vi "GetAccumulationBlockInfo.vi"(9 "block":T4, 10 "start index":i32, 11 "accumulation settings":T1) -> (1 "condition met":bool, 2 "stop index (include)":i32, 3 "updated accumulation settings":T1, 5 "acquired (pulses)":i32, 7 "acquired (sec)":dbl)   [LabVIEW 2017, in "DataAccumulator.lvlib"]
uses:
  <vilib>/addons/InsightCM/Devices/Shared/Common/DataAccumulator/DataAccumulator.lvlib
  <vilib>/addons/InsightCM/Devices/Shared/Common/DataAccumulator/controls/AccumulationSettings.ctl
  <vilib>/addons/InsightCM/Devices/Shared/Common/DataAccumulator/controls/accumulationType.ctl
  <vilib>/addons/InsightCM/Devices/Shared/Common/DVRBuffer/controls/BufferLocation.ctl
  <vilib>/addons/InsightCM/Devices/Shared/Common/DVRBuffer/controls/DVRElement.ctl
  <vilib>/addons/InsightCM/Devices/Shared/Common/DVRBuffer/DVRBuffer.lvlib
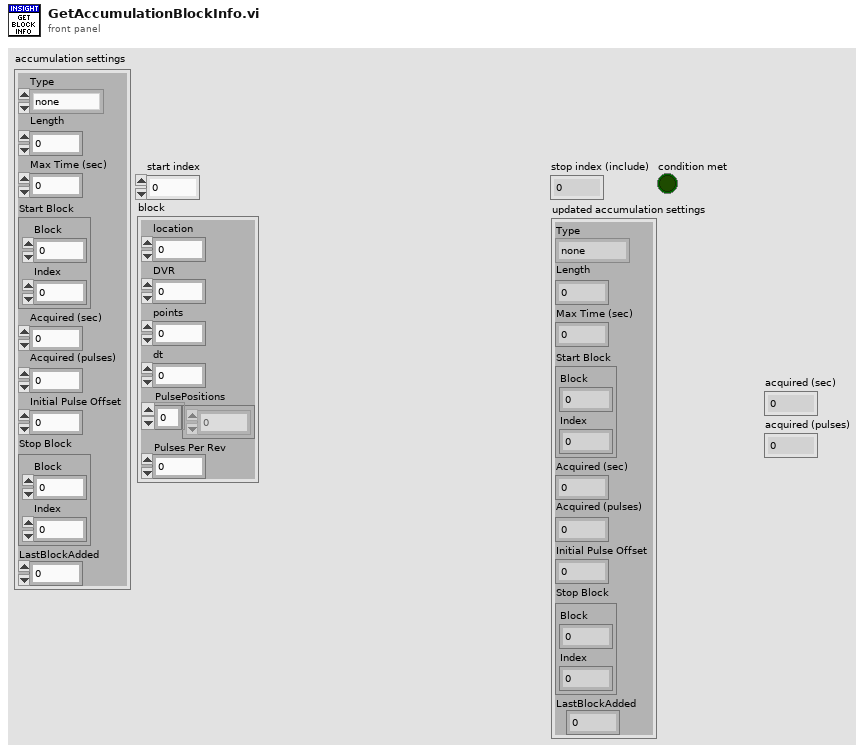
[diagram p1: front panel]
types:
  T1 = typedef "DataAccumulator.lvlib/AccumulationSettings.ctl" = cluster{"Type":T2, "Length":dbl, "Max Time (sec)":dbl, "Start Block":T3, "Acquired (sec)":dbl, "Acquired (pulses)":i32, "Initial Pulse Offset":dbl, "Stop Block":T3, "LastBlockAdded":u32}
  T2 = typedef "DataAccumulator.lvlib/accumulationType.ctl" = enum16{"none", "seconds", "revolutions"}
  T3 = typedef "DVRBuffer.lvlib/BufferLocation.ctl" = cluster{"Block":u32, "Index":i32}
  T4 = typedef "DVRBuffer.lvlib/DVRElement.ctl" = cluster{"location":u32, "DVR":u32, "points":i32, "dt":dbl, "PulsePositions":dbl[], "Pulses Per Rev":dbl}
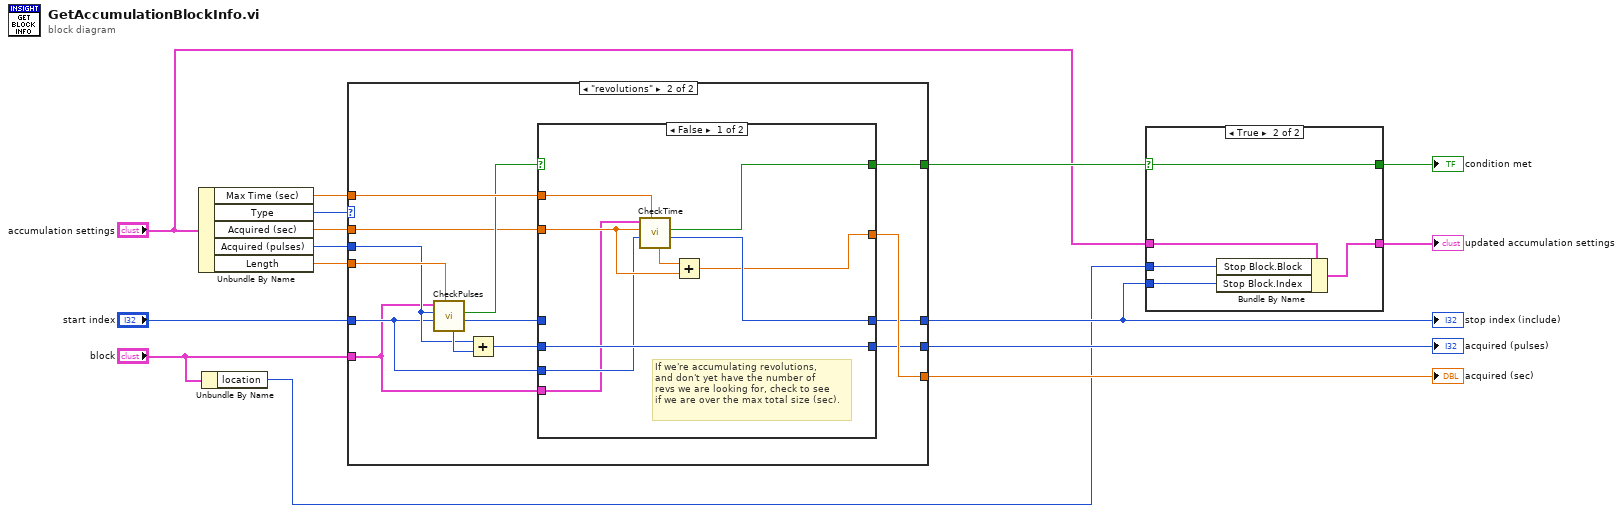
[diagram p0: block diagram]
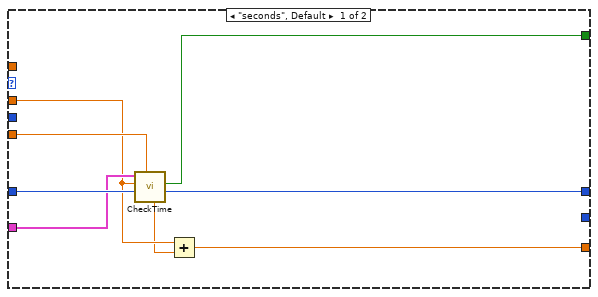
[diagram p3: hidden frame]
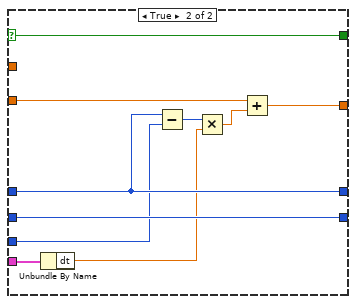
[diagram p4: hidden frame]
diagram:
  n1 = Unbundle By Name("accumulation settings") -> ("Max Time (sec)"=w10:dbl, "Type"=w15:T2, "Acquired (sec)"=w14:dbl, "Acquired (pulses)"=w12:i32, "Length"=w13:dbl)
  n2 = Unbundle By Name("block") -> ("location"=w2:u32)
  n3 = case shown="\"revolutions\"" w15 {
    tunnel: "block" -> [w21 w24]
    tunnel: "start index" -> [w22 w26]
    tunnel: w14 -> [w19 w25]
    tunnel: w13 -> [w20 w37]
    tunnel: [w16 w31] -> w4
    tunnel: [w17 w33] -> w7
    tunnel: [w23 w32] -> w9
    tunnel: w12 -> [_ w35]
    tunnel: w10 -> [_ w34]
    tunnel: [_ w30] -> w8
    frame "seconds", Default {
      n4 = call <vilib>:"CheckTime.vi"("target time"=w20, "start index"=w22, "acquiredSeconds"=w19, "DVR element in"=w21) -> ("stop index (include)"=w16:i32, "time met"=w17:bool, "seconds of data"=w18:dbl)  [unwired: 5 in]
      n5 = Add(x=w19, y=w18) -> (x+y=w23:dbl)
    }
    frame "revolutions" {
      n6 = call <vilib>:"CheckPulses.vi"("target pulses"=w37, "start index"=w26, "acquired pulses in"=w35, "DVR element in"=w24) -> ("stop index (include)"=w27:i32, "pulses met"=w28:bool, "pulses"=w36:i32)  [unwired: 5 in]
      n7 = Add(x=w35, y=w36) -> (x+y=w29:i32)
      n8 = case shown="False" w28 {
        selector: w28 -> [_ w56]
        tunnel: w34 -> [w46 _]
        tunnel: [w45 w56] -> w33
        tunnel: [w41 w52] -> w32
        tunnel: [w44 w51] -> w31
        tunnel: w27 -> [_ w51]
        tunnel: [w43 w55] -> w30
        tunnel: w29 -> [w43 w55]
        tunnel: w26 -> [w39 w50]
        tunnel: w25 -> [w40 w54]
        tunnel: w24 -> [w38 w49]
        frame False {
          # "If we're accumulating revolutions,\nand don't yet have the number of \nrevs we are looking for, check to see\nif we are over the max total size (sec)."
          n9 = call <vilib>:"CheckTime.vi"("target time"=w46, "start index"=w39, "acquiredSeconds"=w40, "DVR element in"=w38) -> ("stop index (include)"=w44:i32, "time met"=w45:bool, "seconds of data"=w42:dbl)  [unwired: 5 in]
          n10 = Add(x=w42, y=w40) -> (x+y=w41:dbl)
        }
        frame True {
          n11 = Unbundle By Name(w49) -> ("dt"=w47:dbl)
          n12 = Subtract(x=w51, y=w50) -> (x-y=w48:i32)
          n13 = Multiply(x=w48, y=w47) -> (x*y=w53:dbl)
          n14 = Add(x=w54, y=w53) -> (x+y=w52:dbl)
        }
      }
    }
  }
  "stop index (include)" <- w4
  "acquired (sec)" <- w9
  "acquired (pulses)" <- w8
  n15 = case shown="True" w7 {
    selector: w7 -> [w58 w63]
    tunnel: [w58 w63] -> w6
    tunnel: [w57 w61] -> w5
    tunnel: "accumulation settings" -> [w57 w62]
    tunnel: w4 -> [_ w60]
    tunnel: w2 -> [_ w59]
    frame False {
    }
    frame True {
      n16 = Bundle By Name(cluster=w62, "Stop Block.Block"=w59, "Stop Block.Index"=w60) -> (w61:T1)
    }
  }
  "updated accumulation settings" <- w5
  "condition met" <- w6
